vi "String to Array Regex.vi"(2 "Regex":string, 3 "Message":string) -> (1 "String to Array":string[](array[string]))   [LabVIEW 2014]
uses:
  <vilib>/regexp/Match Regular Expression.xnode
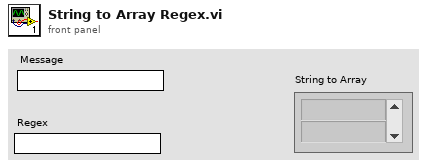
[diagram p1: front panel]
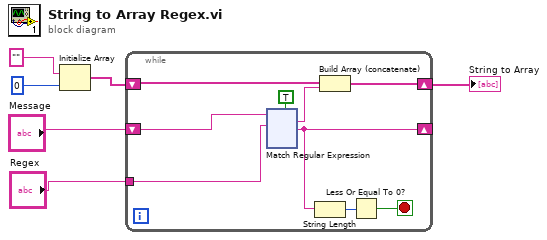
[diagram p0: block diagram]
diagram:
  n1 = Initialize Array("", 0) -> (w4:string[])
  n2 = while {
    shift-right: [w8] -> _
    shift-left: "Message" -> [w11]
    shift-right: [w7] -> w1
    shift-left: w4 -> [w12]
    tunnel: "Regex" -> [w9]
    stop <- w14 stop-if-true
    n3 = xnode "Match Regular Expression"("input string"=w11, "regular expression"=w9, "multiline? (F)"=TRUE) -> ("whole match"=w10:string, "after match"=w8:string)  [unwired: 3 in, 3 out]
    n4 = String Length(string=w8) -> (length=w13:i32)
    n5 = Build Array (concatenate)(w12, w10) -> (w7:string[])
    n6 = Less Or Equal To 0?(x=w13) -> (x <= 0?=w14:bool)
  }
  "String to Array" <- w1
